vi "Lip Outer width SubVI.vi"(0 "Image":T1, 5 "Coord details":T2, 7 "Calibrated Image":T1, 11 "error in (no error)":errorcluster, 12 "M ROI":T4) -> (4 "Image Out":T1, 6 "Lip Outer Width":sgl format="%.2f", 8 "Perpendicular Lines":T3(array[cluster])=[{{"X"=55.0, "Y"=48.0}, {"X"=263.0, "Y"=104.0}}, {{"X"=53.0, "Y"=53.0}, {"X"=262.0, "Y"=109.0}}, {{"X"=52.0, "Y"=58.0}, {"X"=261.0, "Y"=113.0}}, {{"X"=51.0, "Y"=62.0}, {"X"=259.0, "Y"=118.0}}, {{"X"=49.0, "Y"=67.0}, {"X"=258.0, "Y"=123.0}}, {{"X"=48.0, "Y"=72.0}, {"X"=257.0, "Y"=128.0}}, {{"X"=47.0, "Y"=77.0}, {"X"=255.0, "Y"=133.0}}, {{"X"=46.0, "Y"=82.0}, {"X"=254.0, "Y"=138.0}}, {{"X"=44.0, "Y"=87.0}, {"X"=253.0, "Y"=142.0}}, {{"X"=43.0, "Y"=91.0}, {"X"=252.0, "Y"=147.0}}, {{"X"=42.0, "Y"=96.0}, {"X"=250.0, "Y"=152.0}}] {"?"."Y" format="%.2f"; "?"."X" format="%.2f"; "?"."Y" format="%.2f"; "?"."X" format="%.2f"}, 14 "Edge Coordinates":cluster{"X":sgl, "Y":sgl}[](array[cluster]) {"Y" format="%.2f"; "X" format="%.2f"}, 15 "error out":errorcluster)   [LabVIEW 2019, in "Algorithm.lvclass"]
uses:
  FrameworkOverrides/Algorithm.lvclass
  <vilib>/vision/Measure.llb/Edge Polarity.ctl
  <vilib>/vision/Measure.llb/Edge Options.ctl
  <vilib>/vision/Image Controls.llb/IMAQ Image.ctl
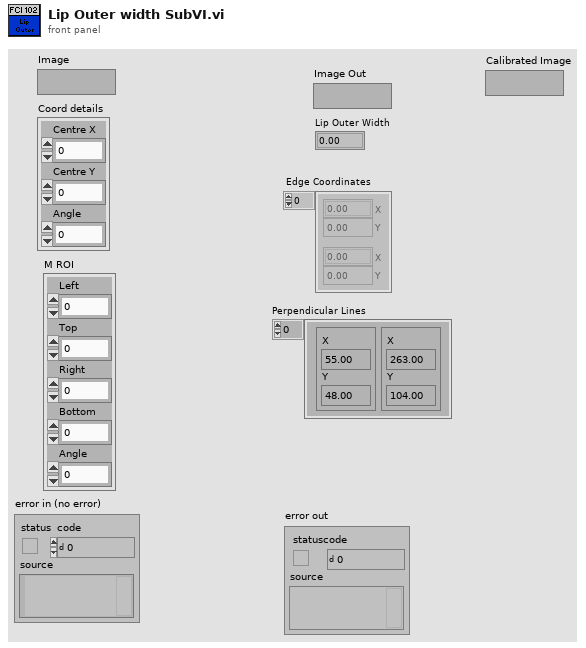
[diagram p1: front panel]
types:
  T1 = typedef "IMAQ Image.ctl" = refnum<image>
  T2 = cluster{"Centre X":dbl, "Centre Y":dbl, "Angle":dbl}
  T3 = cluster{cluster{"X":sgl, "Y":sgl}, cluster{"X":sgl, "Y":sgl}}[]
  T4 = cluster{"Left":dbl, "Top":dbl, "Right":dbl, "Bottom":dbl, "Angle":dbl}
  T5 = typedef "Edge Options.ctl" = cluster{"Edge Polarity":T6, "Kernel Size":u32, "Width":u32, "Minimum Edge Strength":sgl, "Interpolation Type":enum32{"Zero Order", "Bilinear", "Quadratic", "Cubic", "Bilinear Fixed"}, "Data Processing Method":enum32{"Average", "Median"}}
  T6 = typedef "Edge Polarity.ctl" = u32
  T7 = typedef "ROI Descriptor" = cluster{"Global Rectangle":i32[], "Contours":cluster{"ID":enum32{"External", "Internal"}, "Type":u32, "Coordinates":i32[]}[]}
  T8 = typedef "Search Line.ctl" = cluster{"Start Point":cluster{"X":sgl, "Y":sgl}, "End Point":cluster{"X":sgl, "Y":sgl}, "Edge Info":T9[], "Edge Map":dbl[], "Calibration Valid":bool}
  T9 = typedef "Edge New.ctl" = cluster{"Location (Pixel)":cluster{"X":sgl, "Y":sgl}, "Location (Real-World)":cluster{"X":sgl, "Y":sgl}, "Distance (Pixel)":dbl, "Distance (Real-World)":dbl, "Strength":dbl, "Noise":dbl, "Rising?":bool}
  T10 = cluster{"Search Lines":T8[], "First Edge Points Array":cluster{"X":sgl, "Y":sgl}[], "Last Edge Points Array":cluster{"X":sgl, "Y":sgl}[]}
  T11 = cluster{"First Edge Point":cluster{"X":sgl, "Y":sgl}, "Search Line First Edge":cluster{"X":sgl, "Y":sgl}}
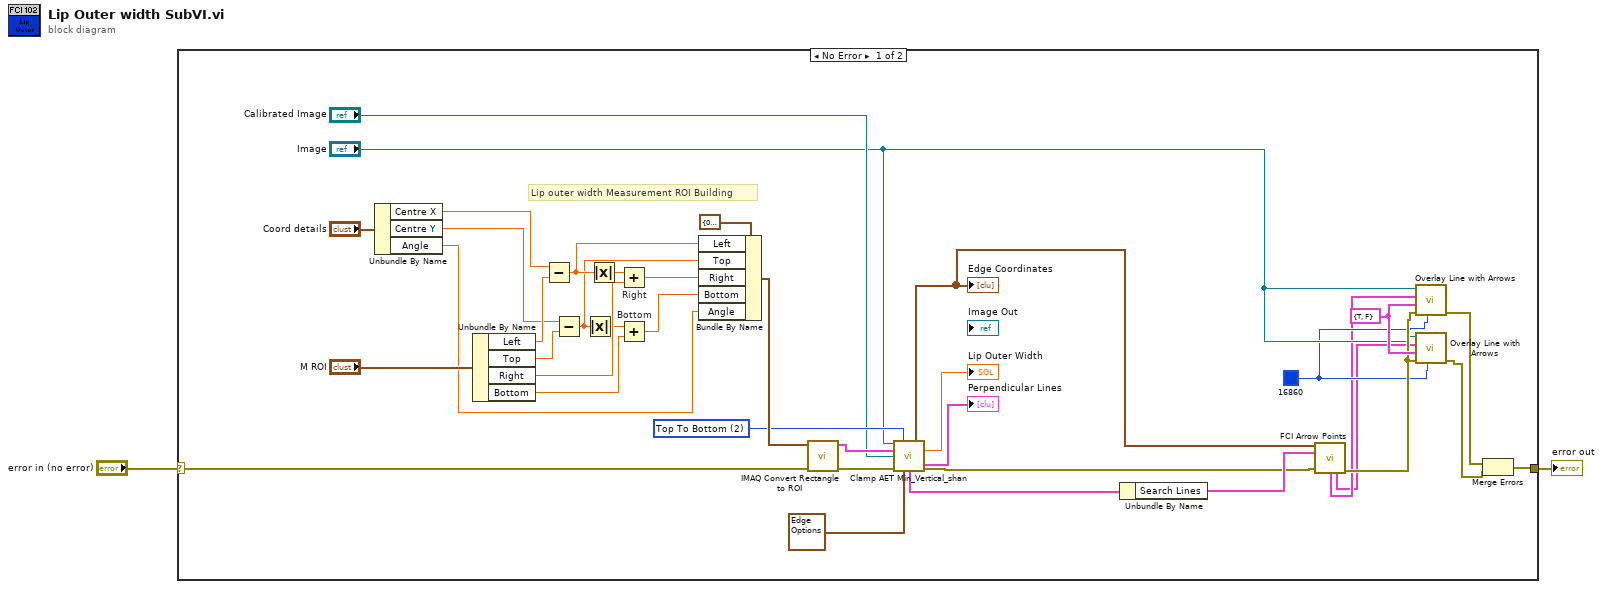
[diagram p0: block diagram]
diagram:
  n1 = case shown="No Error" "error in (no error)" {
    selector: "error in (no error)" -> [w17 w41]
    tunnel: [w6 w41] -> w1
    frame No Error {
      w9 = u32 16860 ("Color")
      w14 = cluster{"Start point":bool, "End point":bool} {"Start point"=TRUE, "End point"=FALSE} ("Arrows")
      w28 = u16 2 items=["Left To Right", "Right To Left", "Top To Bottom", "Bottom To Top"] ("Scanning axis")
      # "Lip outer width Measurement ROI Building"
      n2 = Unbundle By Name("Coord details") -> ("Centre X"=w20:dbl, "Centre Y"=w19:dbl, "Angle"=w18:dbl)
      n3 = Unbundle By Name("M ROI") -> ("Left"=w35:dbl, "Top"=w34:dbl, "Right"=w33:dbl, "Bottom"=w32:dbl)
      n4 = Subtract(x=w20, y=w35) -> (x-y=w38:dbl)
      n5 = Subtract(x=w19, y=w34) -> (x-y=w30:dbl)
      n6 = Absolute Value(x=w30) -> (abs(x)=w31:dbl)
      n7 = Absolute Value(x=w38) -> (abs(x)=w40:dbl)
      n8 = Add "Right"(x=w40, y=w33) -> (x+y=w37:dbl)
      n9 = Add "Bottom"(x=w31, y=w32) -> (x+y=w36:dbl)
      n10 = Bundle By Name(cluster=T4 {"Left"=0.0, "Top"=0.0, "Right"=0.0, "Bottom"=0.0, "Angle"=0.0} ("input cluster"), "Left"=w38, "Top"=w30, "Right"=w37, "Bottom"=w36, "Angle"=w18) -> (w29:T4)
      n11 = call "IMAQ Convert Rectangle to ROI"("error in (no error)"=w17, "Rectangle"=w29) -> ("error out"=w26:errorcluster, "ROI Descriptor"=w24:T7)  [unwired: 7 in]
      n12 = call "Clamp AET Min_Vertical_shan.vi"("Image"="Image", "Scanning axis"=w28, "ROI Descriptor"=w24, "Calibrated Image"="Calibrated Image", "error in (no error)"=w26, "Edge Options"=T5 {"Edge Polarity"=0, "Kernel Size"=3, "Width"=3, "Minimum Edge Strength"=50.0, "Interpolation Type"=enum."Zero Order", "Data Processing Method"=enum."Average"}) -> ("Edge Coordinates"=w5:cluster{"X":sgl, "Y":sgl}[], "Distance"=→"Lip Outer Width":sgl, "Overlay Cluster out"=w11:T10, "Perpendicular Lines"=→"Perpendicular Lines":T3, "error out"=w12:errorcluster)  [unwired: 3 in, 2 out]
      "Edge Coordinates" <- w5
      n13 = Unbundle By Name(w11) -> ("Search Lines"=w15:T8[])
      n14 = call "FCI Arrow Points.vi"("Max Edge Points"=w5, "Search Lines"=w15, "error constant"=w12) -> ("Max first Arrow Line Coord out"=w4:T11, "Max Last Arrow Line Coord out"=w3:T11, "error IO"=w13:errorcluster)  [unwired: 8 in, 2 out]
      n15 = call <vilib>:"Overlay Line with Arrows.vi"("Color"=w9, "error in (no error)"=w13, "Arrows"=w14, "Line Coordinates"=w4, "Image In"="Image") -> ("error out"=w8:errorcluster)  [unwired: 5 in, 1 out]
      n16 = call <vilib>:"Overlay Line with Arrows.vi"("Color"=w9, "error in (no error)"=w13, "Arrows"=w14, "Line Coordinates"=w3, "Image In"="Image") -> ("error out"=w7:errorcluster)  [unwired: 5 in, 1 out]
      n17 = Merge Errors(w8, w7) -> (w6:errorcluster)
    }
    frame Error {
    }
  }
  "error out" <- w1
